vi "frontend_rate.vi"() -> ()   [LabVIEW 2015]
panel:
  out "String 2":string
  out "String":string
  in  "Slide 2":dbl(slide) scale=0.0..100.0
  in  "Slide":dbl(slide) scale=0.0..100.0
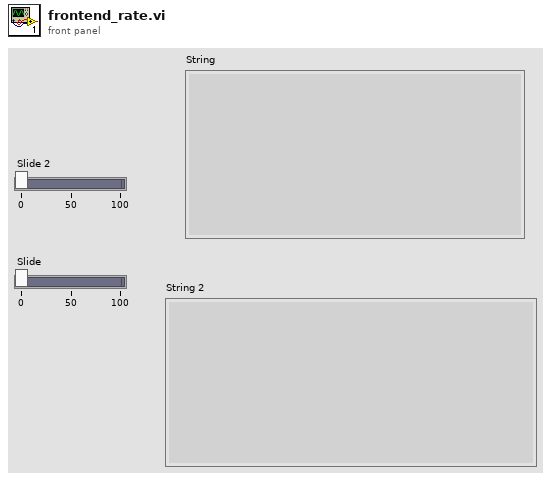
[diagram p1: front panel]
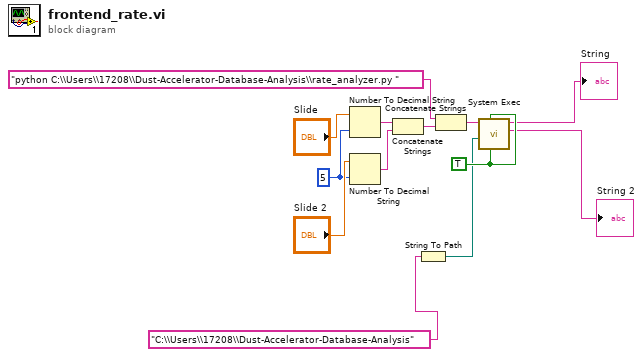
[diagram p0: block diagram]
diagram:
  w5 = TRUE
  w6 = 5
  n1 = Number To Decimal String(number="Slide", width (-)=w6) -> (decimal integer string=w12:string)
  n2 = Number To Decimal String(number="Slide 2", width (-)=w6) -> (decimal integer string=w13:string)
  n3 = Concatenate Strings(w12, w13) -> (w9:string)
  n4 = String To Path(string="C:\\Users\\17208\\Dust-Accelerator-Database-Analysis") -> (path=w1:path)
  n5 = Concatenate Strings("python C:\\Users\\17208\\Dust-Accelerator-Database-Analysis\\rate_analyzer.py ", w9) -> (w7:string)
  n6 = call <vilib>:"System Exec.vi"("run minimized? (F)"=w5, "wait until completion? (T)"=w5, "working directory"=w1, "command line"=w7) -> ("standard error"=→"String 2":string, "standard output"=→"String":string)  [unwired: 4 in, 2 out]
